vi "SLM Control.vi"() -> ()   [LabVIEW 2014]
uses:
  Controls/SLM General Settings.ctl
  Controls/Holo Settings.ctl
  <vilib>/Utility/xml.llb/Write to XML File(string).vi
  <vilib>/Utility/xml.llb/Read From XML File(string).vi
panel:
  in  "Load":bool
  in  "Save":bool
  in  "Exit":bool
  in  "Holo 1 (Doughnut)":T1={"Top Hat"=FALSE, "Modes"=[], "Vortex"=FALSE, "Clockwise"=FALSE, "X"=-200.0, "Y"=0.0, "Holo ON"=TRUE, "Scan"=FALSE} {"Modes"."Amplititute" step=0.05}
  out "Intensity Graph":u8[][](graph)
  in  "Holo 0 (Z)":T1={"Top Hat"=FALSE, "Modes"=[], "Vortex"=FALSE, "Clockwise"=FALSE, "X"=200.0, "Y"=0.0, "Holo ON"=TRUE, "Scan"=FALSE} {"Modes"."Amplititute" step=0.05}
  in  "General settings":T2={"Holo size (pixels)"=300, "Top hat radius"=0.5, "Number of modes"=20, "Bkg gradient X"=40.0, "Bkg gradient Y"=40.0, "Flat"=FALSE, "Mode Matrix"=1} {"Mode Matrix" items=["Unit Matrix", "Unit Matrix_AbbNames"]; "Top hat radius" min=0.0 max=0.99 step=0.05 format="%.3f"}
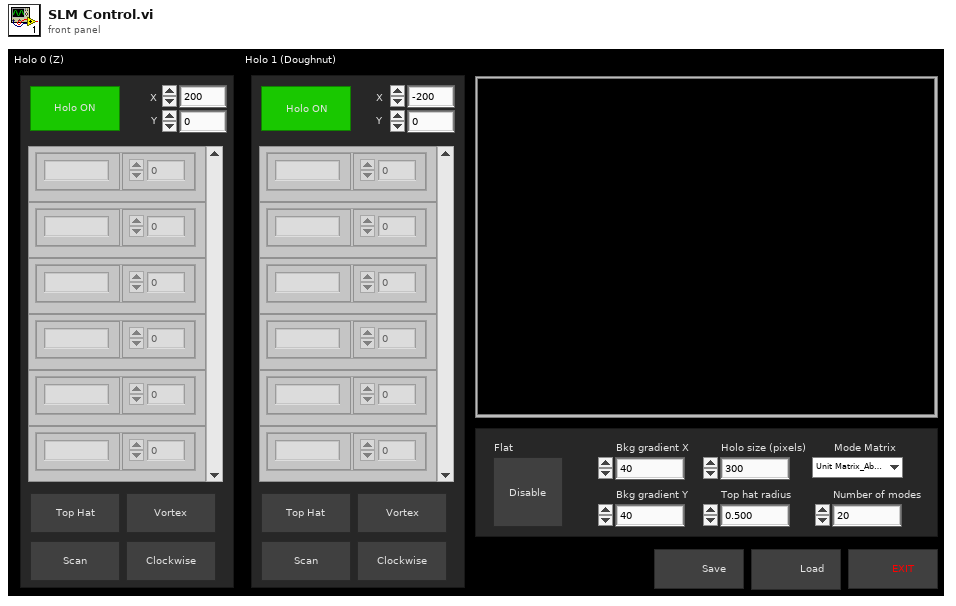
[diagram p1: front panel]
types:
  T1 = typedef "Holo Settings.ctl" = cluster{"Top Hat":bool, "Modes":cluster{"Mode ID":string, "Amplititute":dbl}[], "Vortex":bool, "Clockwise":bool, "X":dbl, "Y":dbl, "Holo ON":bool, "Scan":bool}
  T2 = typedef "SLM General Settings.ctl" = cluster{"Holo size (pixels)":i32, "Top hat radius":dbl, "Number of modes":i32, "Bkg gradient X":dbl, "Bkg gradient Y":dbl, "Flat":bool, "Mode Matrix":u16}
  T3 = cluster{"Holo size (pixels)":bool, "Top hat radius":bool, "Number of modes":bool, "Bkg gradient X":bool, "Bkg gradient Y":bool, "Flat":bool, "Mode Matrix":bool}
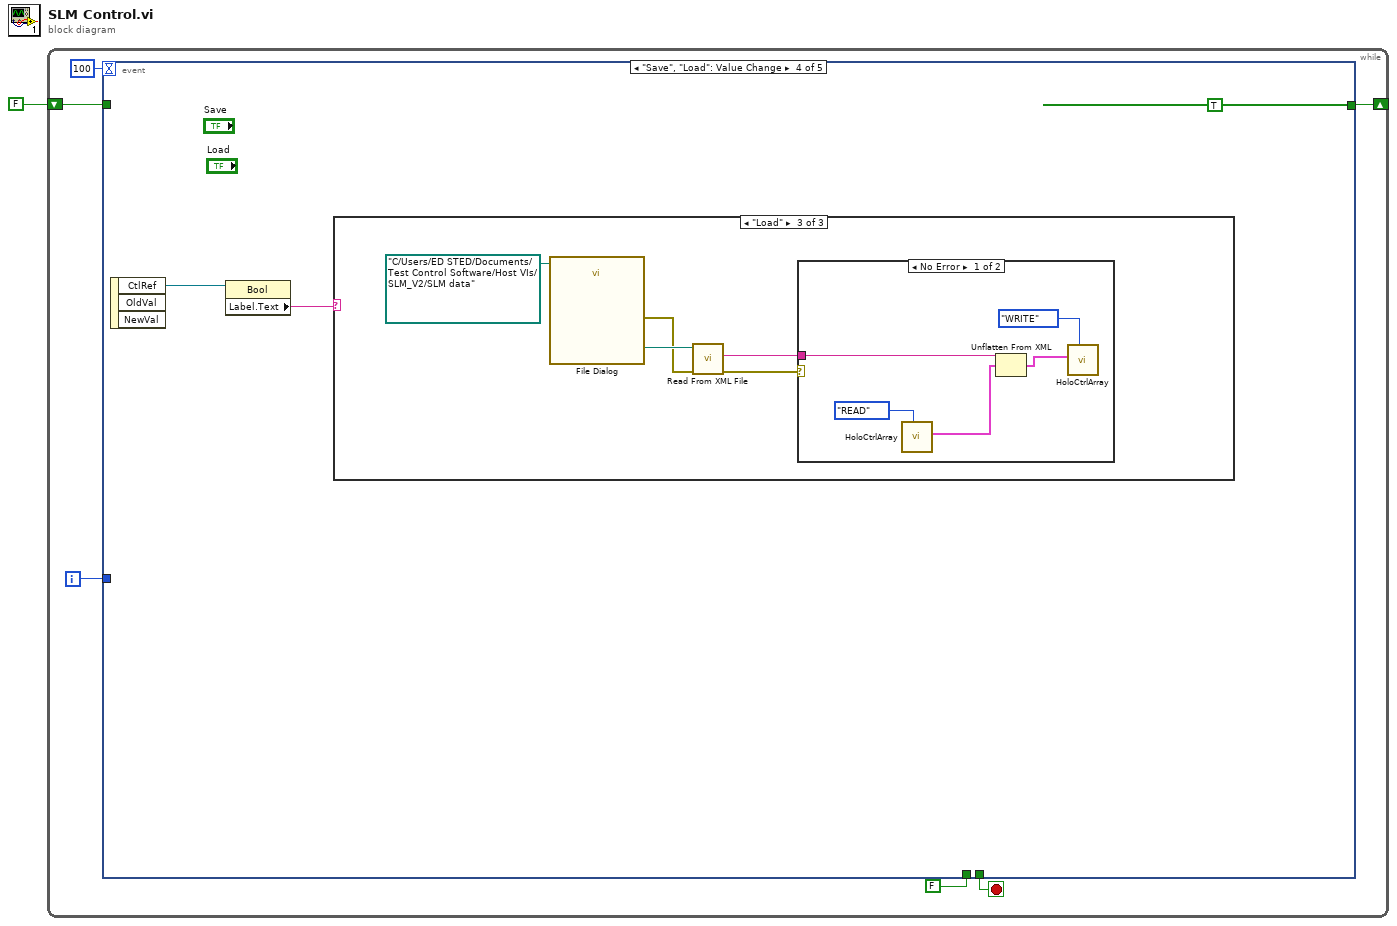
[diagram p0: block diagram]
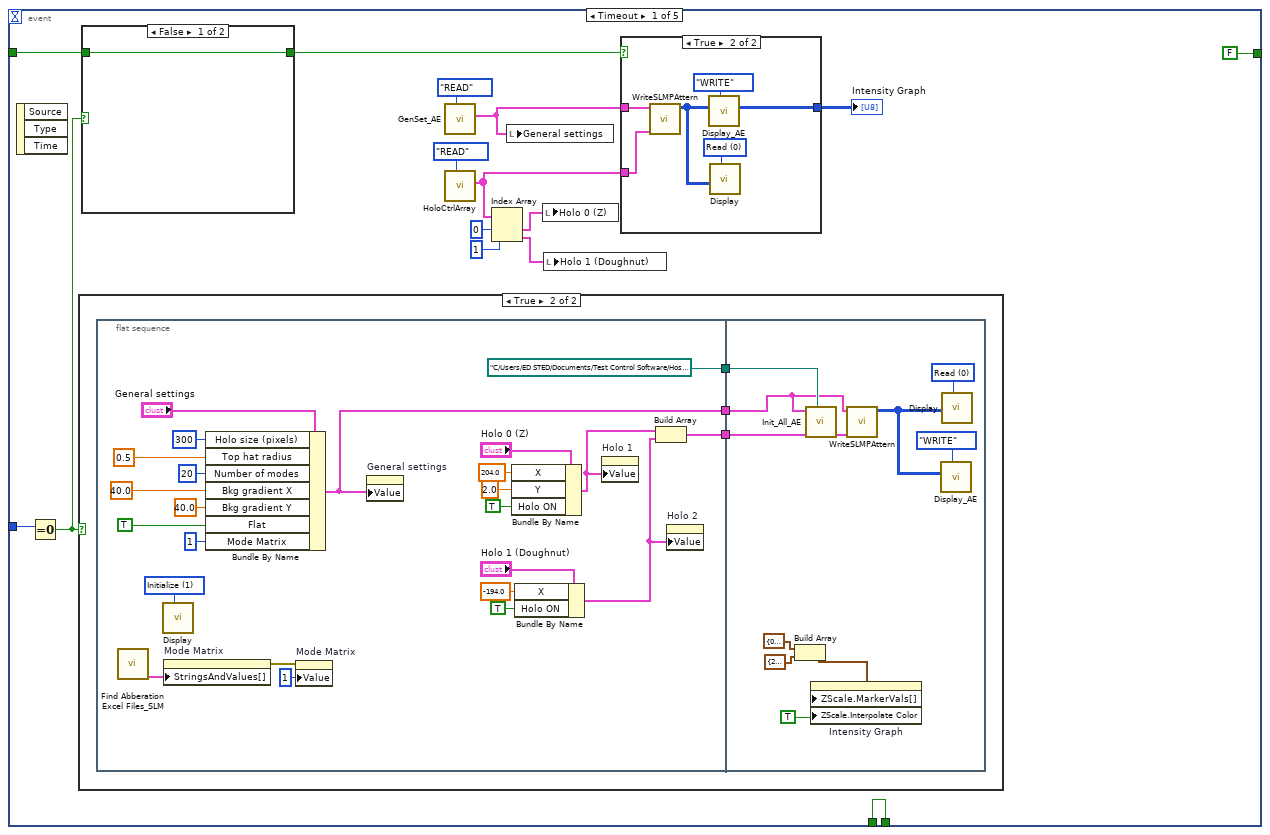
[diagram p2: hidden frame]
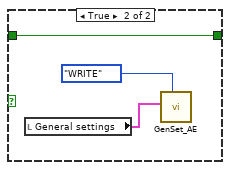
[diagram p3: hidden frame]
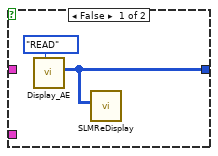
[diagram p4: hidden frame]
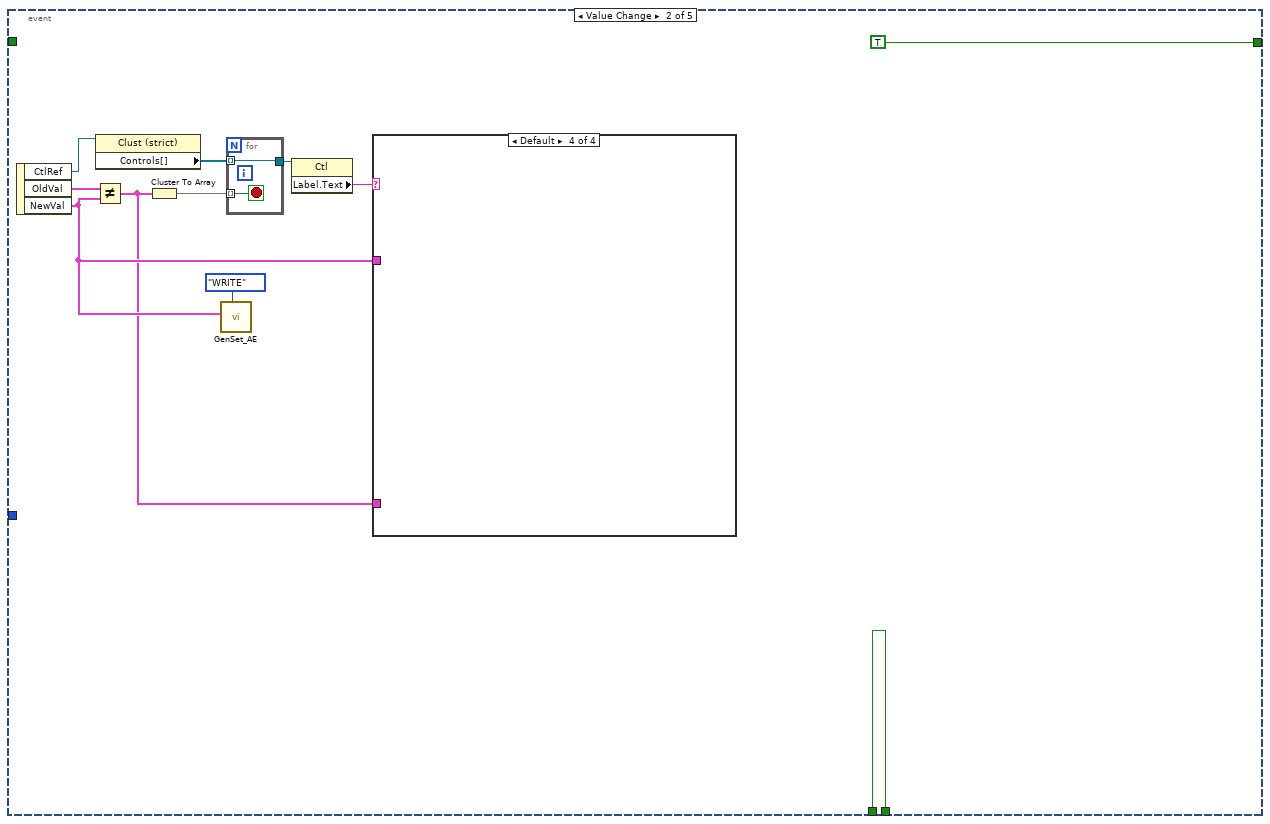
[diagram p6: hidden frame]
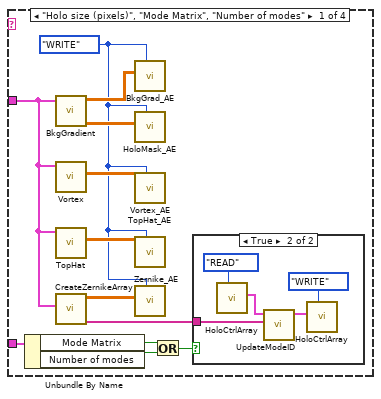
[diagram p7: hidden frame]
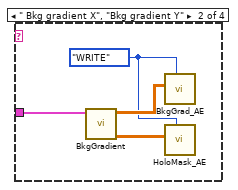
[diagram p9: hidden frame]
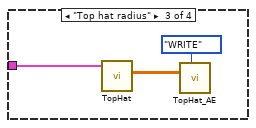
[diagram p10: hidden frame]
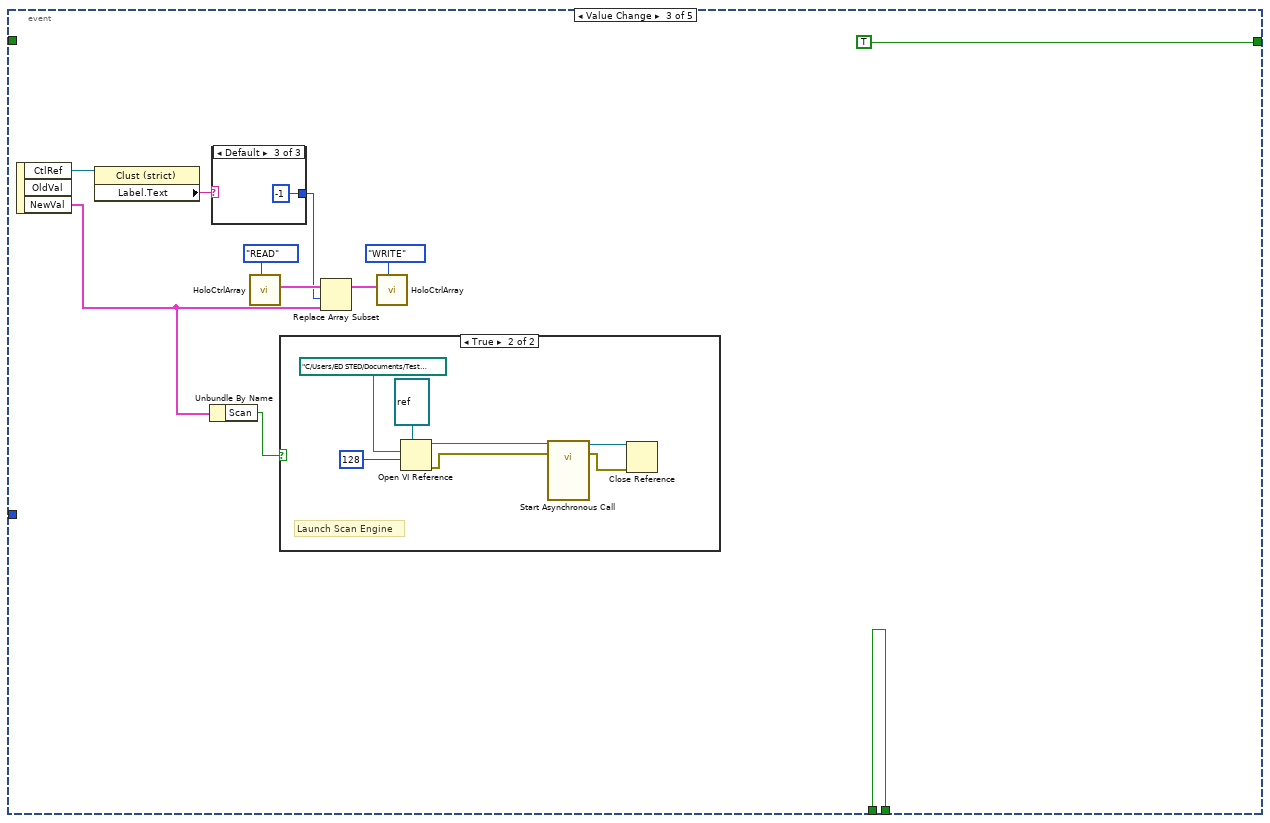
[diagram p11: hidden frame]
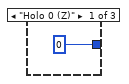
[diagram p13: hidden frame]
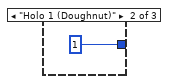
[diagram p14: hidden frame]
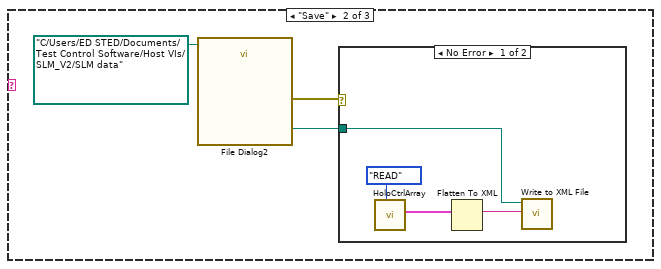
[diagram p16: hidden frame]
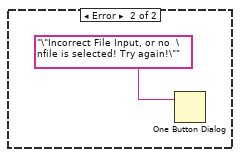
[diagram p17: hidden frame]
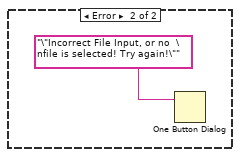
[diagram p18: hidden frame]
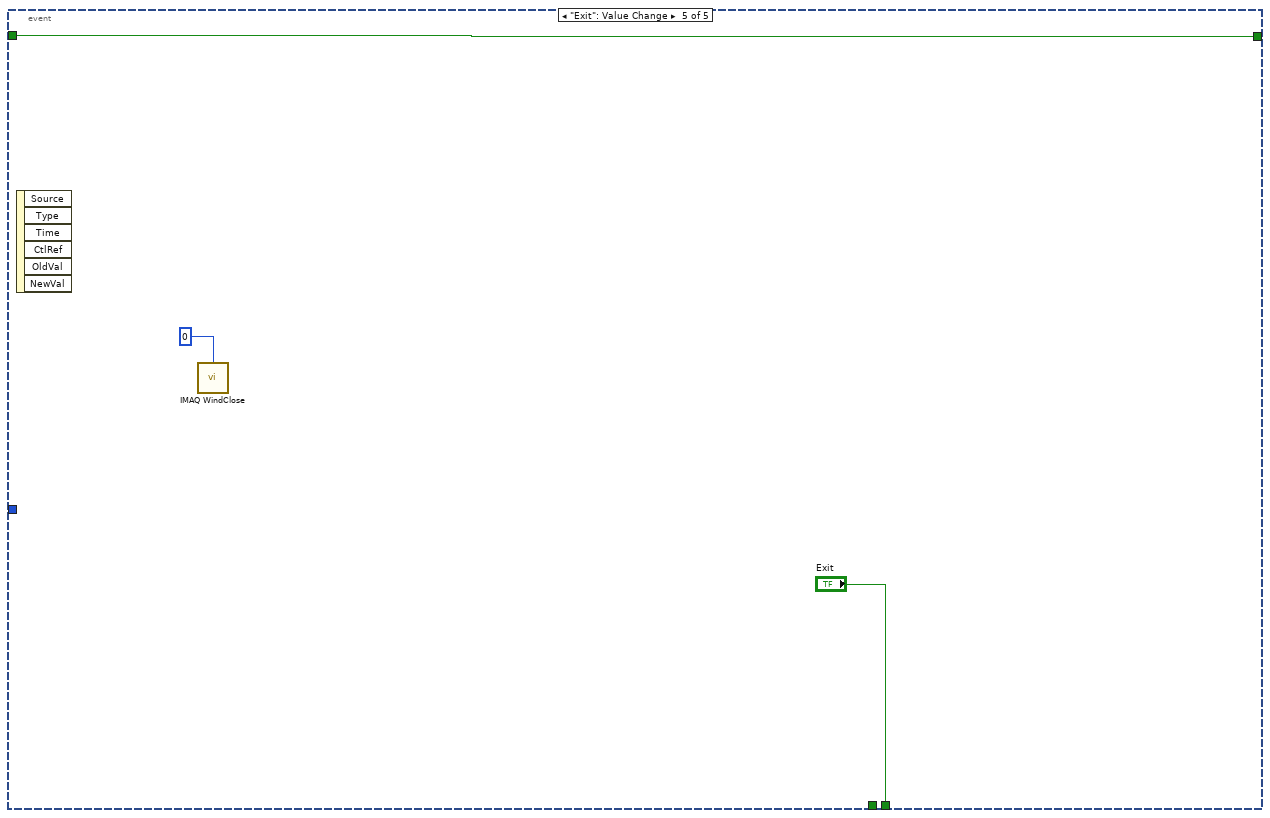
[diagram p19: hidden frame]
diagram:
  n1 = while {
    shift-right: [w4] -> _
    shift-left: FALSE -> [w5]
    i -> [w6]
    stop <- w3 stop-if-true
    n2 = event shown="[3] \"Save\", \"Load\": Value Change" {
      selector: _ -> [_ _ _ _ _]
      dyn-events: _ -> [_ _ _ _ _]
      timeout: 100 -> [_ _ _ _ _]
      tunnel: w6 -> [w22 _ _ _ _]
      tunnel: w5 -> [w10 _ _ _ w154]
      tunnel: [FALSE TRUE TRUE TRUE w154] -> w4
      tunnel: [w11 w74 w112 _ "Exit"] -> w3
      tunnel: FALSE -> [w11 w74 w112 _ _]
      event Timeout {
        n3 = event-data() -> ()  [unwired: 1 in, 3 out]
        n4 = Equal To 0?(x=w22) -> (x = 0?=w8:bool)
        n5 = case shown="True" w8 {
          frame False {
          }
          frame True {
            n6 = flat-sequence {
              tunnel: [w41] -> w37
              tunnel: [w57] -> w36
              tunnel: [path "C:/Users/ED STED/Documents/Test Control Software/Host VIs/SLM_V2/Flatness Correction LSH0701019/CAL_LSH0701019_770nm.bmp" ("Flat File Path")] -> w35
              tunnel: w37 -> [w64]
              tunnel: w36 -> [w72]
              tunnel: w35 -> [w69]
              frame #0 {
                w58 = u16 1 items=["Read", "Initialize"] ("Action")
                n7 = call "Find Abberation Excel Files_SLM.vi"() -> ("Ring Menu"=w61:cluster{"result string":string, i32}[])  [unwired: 10 in, 1 out]
                n8 = call "Display.vi"("Action"=w58) -> ()  [unwired: 10 in, 1 out]
                n9 = property on="Mode Matrix" class="Ring (strict)"("StringsAndValues[]"=w61) -> (error out=w60:errorcluster)  [unwired: 2 in, 1 out]
                n10 = Bundle By Name(cluster="General settings", "Holo size (pixels)"=300, "Top hat radius"=0.5, "Number of modes"=20, "Bkg gradient X"=40.0, "Bkg gradient Y"=40.0, "Flat"=TRUE, "Mode Matrix"=u16 1) -> (w41:T2)
                n11 = property on="Mode Matrix" class="Ring (strict)"(error in=w60, "Value"=u16 1) -> ()  [unwired: 1 in, 2 out]
                n12 = property on="General settings" class="Clust (strict)"("Value"=w41) -> ()  [unwired: 2 in, 2 out]
                n13 = Bundle By Name(cluster="Holo 0 (Z)", "X"=204.0, "Y"=2.0, "Holo ON"=TRUE) -> (w45:T1)
                n14 = Bundle By Name(cluster="Holo 1 (Doughnut)", "X"=-194.0, "Holo ON"=TRUE) -> (w42:T1)
                n15 = property on="Holo 1" class="Clust (strict)"("Value"=w45) -> ()  [unwired: 2 in, 2 out]
                n16 = Build Array(w45, w42) -> (w57:T1[])
                n17 = property on="Holo 2" class="Clust (strict)"("Value"=w42) -> ()  [unwired: 2 in, 2 out]
              }
              frame #1 {
                w71 = u16 0 items=["Read", "Initialize"] ("Action")
                n18 = Build Array(cluster{dbl, u32} {0.0, 0}, cluster{dbl, u32} {255.0, 16448250}) -> (w65:cluster{dbl, u32}[])
                n19 = call "Init_All_AE.vi"("Flat File Path"=w69, "HoloArray In"=w72, "General settings"=w64) -> ("Holo Array Out"=w70:T1[])  [unwired: 8 in]
                n20 = property on="Intensity Graph" class="IntGraph (strict)"("ZScale.MarkerVals[]"=w65, "ZScale.Interpolate Color"=TRUE ("Z Scale.Interpolate Color")) -> ()  [unwired: 2 in, 2 out]
                n21 = call "WriteSLMPAttern.vi"("Holo Array"=w70, "General settings"=w64) -> ("Display Array"=w62:u8[][])  [unwired: 9 in]
                n22 = call "Display_AE.vi"("Action"=enum16{"READ", "WRITE"}."WRITE", "Display Array In"=w62) -> ()  [unwired: 9 in, 1 out]
                n23 = call "Display.vi"("Action"=w71, "displayed matrix"=w62) -> ()  [unwired: 9 in, 1 out]
              }
            }
          }
        }
        n24 = case shown="False" w8 {
          tunnel: w10 -> [w23 w26]
          tunnel: [w23 w26] -> w9
          frame False {
          }
          frame True {
            n25 = local read "General settings"() -> (w24:T2)
            n26 = call "GenSet_AE.vi"("Enum"=enum16{"READ", "WRITE"}."WRITE", "General settings"=w24) -> ()  [unwired: 9 in, 1 out]
          }
        }
        n27 = call "GenSet_AE.vi"("Enum"=enum16{"READ", "WRITE"}."READ") -> ("General settings Out"=w18:T2)  [unwired: 10 in]
        n28 = call "HoloCtrlArray.vi"("Action"=enum16{"READ", "WRITE"}."READ") -> ("Holo Array Out"=w17:T1[])  [unwired: 10 in]
        n29 = Index Array(array=w17, index #1=0 ("index"), index #2=1 ("index")) -> (element #1=w16:T1, element #2=w15:T1)
        n30 = local write "General settings"(w18) -> ()
        n31 = local write "Holo 0 (Z)"(w16) -> ()
        n32 = local write "Holo 1 (Doughnut)"(w15) -> ()
        n33 = case shown="True" w9 {
          tunnel: w18 -> [_ w34]
          tunnel: w17 -> [_ w33]
          tunnel: [w27 w29] -> w12
          frame False {
            n34 = call "Display_AE.vi"("Action"=enum16{"READ", "WRITE"}."READ") -> ("Display Array Out"=w27:u8[][])  [unwired: 10 in]
            n35 = call "SLMReDisplay.vi"("displayed matrix"=w27) -> ()  [unwired: 11 in]
          }
          frame True {
            w32 = u16 0 items=["Read", "Initialize"] ("Action")
            n36 = call "WriteSLMPAttern.vi"("Holo Array"=w33, "General settings"=w34) -> ("Display Array"=w31:u8[][])  [unwired: 9 in]
            n37 = call "Display_AE.vi"("Action"=enum16{"READ", "WRITE"}."WRITE", "Display Array In"=w31) -> ("Display Array Out"=w29:u8[][])  [unwired: 9 in]
            n38 = call "Display.vi"("Action"=w32, "displayed matrix"=w31) -> ()  [unwired: 9 in, 1 out]
          }
        }
        "Intensity Graph" <- w12
      }
      event Value Change {
        n39 = event-data() -> ("CtlRef"=w82:refnum<vi>, "OldVal"=w83:T2, "NewVal"=w75:T2)  [unwired: 1 in]
        n40 = Not Equal?(x=w83, y=w75) -> (x != y?=w73:T3)
        n41 = property class="Clust (strict)"(reference=w82) -> ("Controls[]"=w81:refnum<vi>[])  [unwired: 1 in, 2 out]
        n42 = Cluster To Array(cluster=w73) -> (array=w80:bool[])
        n43 = call "GenSet_AE.vi"("Enum"=enum16{"READ", "WRITE"}."WRITE", "General settings"=w75) -> ()  [unwired: 9 in, 1 out]
        n44 = for {
          tunnel: [w109] -> w79
          tunnel: w81 -> [w109] mode=indexing
          tunnel: w80 -> [w108] mode=indexing
          stop <- w108 stop-if-true
        }
        n45 = property class="Ctl"(reference=w79) -> ("Label.Text"=w78:string)  [unwired: 1 in, 2 out]
        n46 = case shown="Default" w78 {
          tunnel: w75 -> [w89 w101 w107 _]
          tunnel: w73 -> [w87 _ _ _]
          frame "Holo size (pixels)", "Mode Matrix", "Number of modes" {
            w88 = enum16{"READ", "WRITE"}."WRITE" ("Action")
            n47 = Unbundle By Name(w87) -> ("Mode Matrix"=w86:bool, "Number of modes"=w85:bool)
            n48 = call "BkgGradient.vi"("General settings"=w89) -> ("Holo mask"=w94:dbl[][], "gradient"=w95:dbl[][])  [unwired: 9 in]
            n49 = call "Vortex.vi"("General settings"=w89) -> ("Vortex"=w92:dbl[][])  [unwired: 10 in]
            n50 = call "TopHat.vi"("General settings"=w89) -> ("TopHat"=w93:dbl[][])  [unwired: 10 in]
            n51 = call "CreateZernikeArray.vi"("General settings"=w89) -> ("Mode IDs"=w90:string[], "Modes Out"=w91:dbl[][][])  [unwired: 9 in]
            n52 = call "BkgGrad_AE.vi"("Action"=w88, "BkgGrad In"=w95) -> ()  [unwired: 9 in, 1 out]
            n53 = call "HoloMask_AE.vi"("Action"=w88, "HoloMask In"=w94) -> ()  [unwired: 9 in, 1 out]
            n54 = call "Vortex_AE.vi"("Action"=w88, "Vortex In"=w92) -> ()  [unwired: 9 in, 1 out]
            n55 = call "TopHat_AE.vi"("Action"=w88, "TopHat In"=w93) -> ()  [unwired: 9 in, 1 out]
            n56 = call "Zernike_AE.vi"("Action"=w88, "Zernike In"=w91) -> ()  [unwired: 9 in, 1 out]
            n57 = Or(x=w86, y=w85) -> (x .or. y?=w84:bool)
            n58 = case shown="True" w84 {
              tunnel: w90 -> [_ w100]
              frame False {
              }
              frame True {
                n59 = call "HoloCtrlArray.vi"("Action"=enum16{"READ", "WRITE"}."READ") -> ("Holo Array Out"=w99:T1[])  [unwired: 10 in]
                n60 = call "UpdateModeID.vi"("Mode IDs"=w100, "Array in"=w99) -> ("Array out"=w96:T1[])  [unwired: 9 in]
                n61 = call "HoloCtrlArray.vi"("Action"=enum16{"READ", "WRITE"}."WRITE", "Holo Array In"=w96) -> ()  [unwired: 9 in, 1 out]
              }
            }
          }
          frame " Bkg gradient X", "Bkg gradient Y" {
            w102 = enum16{"READ", "WRITE"}."WRITE" ("Action")
            n62 = call "BkgGradient.vi"("General settings"=w101) -> ("Holo mask"=w103:dbl[][], "gradient"=w104:dbl[][])  [unwired: 9 in]
            n63 = call "BkgGrad_AE.vi"("Action"=w102, "BkgGrad In"=w104) -> ()  [unwired: 9 in, 1 out]
            n64 = call "HoloMask_AE.vi"("Action"=w102, "HoloMask In"=w103) -> ()  [unwired: 9 in, 1 out]
          }
          frame "Top hat radius" {
            n65 = call "TopHat.vi"("General settings"=w107) -> ("TopHat"=w106:dbl[][])  [unwired: 10 in]
            n66 = call "TopHat_AE.vi"("Action"=enum16{"READ", "WRITE"}."WRITE", "TopHat In"=w106) -> ()  [unwired: 9 in, 1 out]
          }
          frame Default {
          }
        }
      }
      event Value Change {
        n67 = event-data() -> ("CtlRef"=w117:refnum<vi>, "NewVal"=w111:T1)  [unwired: 1 in, 1 out]
        n68 = property class="Clust (strict)"(reference=w117) -> ("Label.Text"=w116:string)  [unwired: 1 in, 2 out]
        n69 = Unbundle By Name(w111) -> ("Scan"=w110:bool)
        n70 = case shown="Default" w116 {
          tunnel: [0 1 -1] -> w115
          frame "Holo 0 (Z)" {
          }
          frame "Holo 1 (Doughnut)" {
          }
          frame Default {
          }
        }
        n71 = call "HoloCtrlArray.vi"("Action"=enum16{"READ", "WRITE"}."READ") -> ("Holo Array Out"=w118:T1[])  [unwired: 10 in]
        n72 = case shown="True" w110 {
          frame False {
          }
          frame True {
            # "Launch Scan Engine"
            n73 = Open VI Reference(type specifier VI Refnum (for type only)=refnum<vi> refnum, vi path=path "C:/Users/ED STED/Documents/Test Control Software/Host VIs/SLM_V2/Scan/ScanMode_SLM.vi", options=128) -> (vi reference=w122:refnum<vi>, error out=w121:errorcluster)  [unwired: 3 in]
            n74 = call-by-ref "Start Asynchronous Call"(reference=w122, error in=w121) -> (reference out=w124:refnum<vi>, error out=w123:errorcluster)  [unwired: 12 in]
            n75 = Close Reference(reference=w124, error in (no error)=w123) -> ()  [unwired: 1 out]
          }
        }
        n76 = Replace Array Subset(array=w118, new element=w111, index=w115) -> (w113:T1[])
        n77 = call "HoloCtrlArray.vi"("Action"=enum16{"READ", "WRITE"}."WRITE", "Holo Array In"=w113) -> ()  [unwired: 9 in, 1 out]
      }
      event "Save", "Load": Value Change {
        n78 = event-data() -> ("CtlRef"=w133:refnum<vi>)  [unwired: 1 in, 2 out]
        n79 = property class="Bool"(reference=w133) -> ("Label.Text"=w132:string)  [unwired: 1 in, 2 out]
        n80 = case shown="\"Load\"" w132 {
          frame Default {
          }
          frame "Save" {
            n81 = call "File Dialog2"("start path"=path "C:/Users/ED STED/Documents/Test Control Software/Host VIs/SLM_V2/SLM data") -> ("selected path"=w135:path, "error out"=w134:errorcluster)  [unwired: 11 in, 2 out]
            n82 = case shown="No Error" w134 {
              tunnel: w135 -> [w137 _]
              frame No Error {
                n83 = call "HoloCtrlArray.vi"("Action"=enum16{"READ", "WRITE"}."READ") -> ("Holo Array Out"=w139:T1[])  [unwired: 10 in]
                n84 = Flatten To XML(anything=w139) -> (xml string=w138:string)
                n85 = call-poly <vilib>:"Write to XML File.vi"("XML Input"=w138, "XML File Path"=w137) -> ()  [unwired: 7 in, 3 out]
              }
              frame Error {
                n86 = One Button Dialog(message="\"Incorrect File Input, or no  \nfile is selected! Try again!\"") -> ()  [unwired: 1 in, 1 out]
              }
            }
          }
          frame "Load" {
            n87 = call "File Dialog"("start path"=path "C:/Users/ED STED/Documents/Test Control Software/Host VIs/SLM_V2/SLM data") -> ("selected path"=w145:path, "error out"=w142:errorcluster)  [unwired: 11 in, 2 out]
            n88 = call-poly <vilib>:"Read From XML File.vi"("error in (no error)"=w142, "XML File Path"=w145) -> ("error out"=w143:errorcluster, "XML Elements"=w146:string)  [unwired: 7 in, 1 out]
            n89 = case shown="No Error" w143 {
              tunnel: w146 -> [w151 _]
              frame No Error {
                n90 = call "HoloCtrlArray.vi"("Action"=enum16{"READ", "WRITE"}."READ") -> ("Holo Array Out"=w149:T1[])  [unwired: 10 in]
                n91 = Unflatten From XML(xml string=w151, type=w149) -> (value=w148:T1[])  [unwired: 1 in, 1 out]
                n92 = call "HoloCtrlArray.vi"("Action"=enum16{"READ", "WRITE"}."WRITE", "Holo Array In"=w148) -> ()  [unwired: 9 in, 1 out]
              }
              frame Error {
                n93 = One Button Dialog(message="\"Incorrect File Input, or no  \nfile is selected! Try again!\"") -> ()  [unwired: 1 in, 1 out]
              }
            }
          }
        }
      }
      event "Exit": Value Change {
        n94 = event-data() -> ()  [unwired: 1 in, 6 out]
        n95 = call "IMAQ WindClose"("Window Number (0...15)"=0) -> ()  [unwired: 2 in, 4 out]
      }
    }
  }
